vi "Remote Tasp.vi"(3 "Rack":u16, 5 "Slot":u16) -> (1 "RemoteTSAP":i16)   [LabVIEW 2014, in "Simatic S7.lvlib"]
uses:
  Simatic S7.lvlib
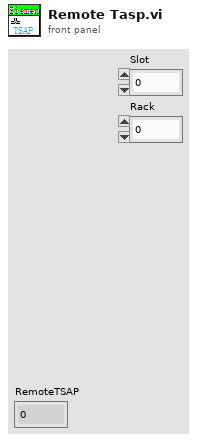
[diagram p1: front panel]
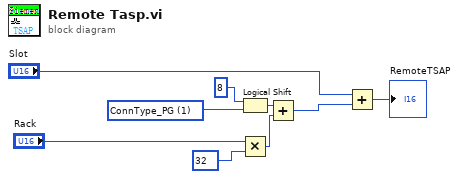
[diagram p0: block diagram]
diagram:
  w8 = u16 1 items=["ConnType_PG"=1, "ConnType_OP"=2, "ConnType_BASIC"=3] ("ConnType")
  n1 = Logical Shift(y=u16 8 ("x"), x=w8) -> (x << y=w7:u16)
  n2 = Multiply(x="Rack", y=i16 32) -> (x*y=w5:u16)
  n3 = Add(x=w7, y=w5) -> (x+y=w4:u16)
  n4 = Add(x="Slot", y=w4) -> (x+y=→"RemoteTSAP":u16)
